vi "Match Array of Patterns.vi"(8 "Patterns":string[](array[string]), 10 "String":string) -> (0 "Index of element":i32, 2 "Found?":bool)   [LabVIEW 2017, in "XTree.xctl"]
doc: "Compares a string against an array of regular expressions. If a match is found, the index will be returned, otherwise it will return -1."
uses:
  <vilib>/addons/_NIFileIO/XTree/XTree.xctl
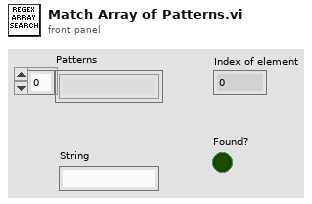
[diagram p1: front panel]
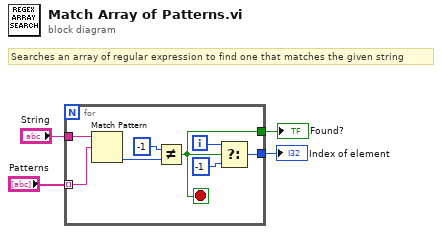
[diagram p0: block diagram]
diagram:
  # "Searches an array of regular expression to find one that matches the given string"
  n1 = for {
    tunnel: "Patterns" -> [w10] mode=indexing
    tunnel: "String" -> [w9]
    tunnel: [w6] -> w2
    tunnel: [w5] -> w1
    i -> [w8]
    stop <- w5 stop-if-true
    n2 = Match Pattern(string=w9, regular expression=w10) -> (offset past match=w12:i32)  [unwired: 1 in, 3 out]
    n3 = Not Equal?(x=-1 ("y"), y=w12) -> (x != y?=w5:bool)
    n4 = Select(t=w8, s=w5, f=-1 ("Index of element")) -> (s? t:f=w6:i32)
  }
  "Index of element" <- w2
  "Found?" <- w1
